vi "Name.vi"(8 "error in (no error)":errorcluster, 11 "LUnit Test Case in":refnum<class "LUnit Inheriting Test Case.lvclass">) -> (0 "error out":errorcluster, 2 "Name":string, 3 "LUnit Test Case out":refnum<class "LUnit Inheriting Test Case.lvclass">)   [LabVIEW 2020]
uses:
  LUnit Inheriting Test Case.lvclass
  LUnit Inheriting Test Case.lvclass/LUnit Inheriting Test Case.ctl
  C:/git/astemes-lunit/source/API/LUnit Test Case/LUnit Test Case.lvclass
  C:/git/astemes-lunit/source/Core/Runnable/Runnable.lvclass
  C:/git/astemes-lunit/source/API/LUnit Inheriting Test Case/LUnit Test Case/LUnit Inheriting Test Case.lvclass
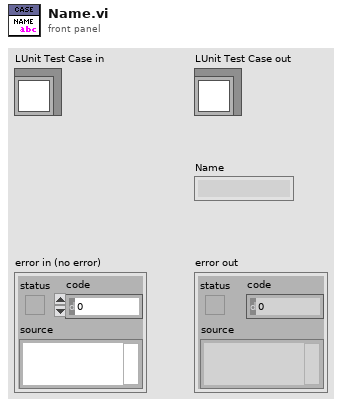
[diagram p1: front panel]
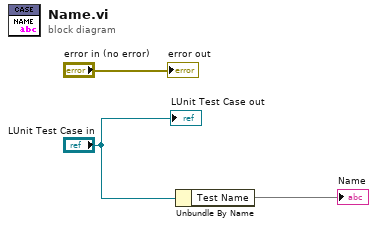
[diagram p0: block diagram]
diagram:
  n1 = Unbundle By Name("LUnit Test Case in") -> ("Test Name"=→"Name")
  "error out" <- "error in (no error)"
  "LUnit Test Case out" <- "LUnit Test Case in"
